vi "TPG361_Global.vi"() -> ()   [LabVIEW 2019]
panel:
  out "TPG361_ST":u32(colorbox)
  out "TPG361_p":dbl
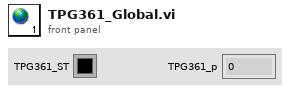
[diagram p1: front panel]
diagram:
